vi "(SubVI)Scope_Log with Trigger.vi"(4 "Sampling Time":dbl format="%#_13g", 5 "Channel Settings":T1[](array[typedef]) {"Address" format="%04x"}, 6 "Log File Length":dbl=1.0 caption="Log File Length (sec.)" min=1.0, 7 "Init":bool, 8 "error in (no error)":errorcluster caption="에러 입력(에러 없음)", 9 "Trigger Setting":T2 {"Capture Delay (sec.)" min=0.0 max=5.0; "Pre-Trigger (sec.)" max=10.0}, 10 "Scope Data In":i16[][](array[numeric]), 11 "Path":path) -> (0 "error out":errorcluster caption="에러 출력", 3 "File Ref Out":refnum<file>)   [LabVIEW 2020]
uses:
  Controls/(Ctrl)Scope_Log_Trigger_Setting.ctl
  Controls/(Ctrl)Scope_Log_Trigger_Type.ctl
  Controls/(Ctrl)Scope_Log_Trigger_Edge.ctl
  Controls/(Ctrl)Scope_Log_Trigger_Edge_Slope.ctl
  Controls/(Ctrl)Scope_Log_Trigger_Window.ctl
  Controls/(Ctrl)Scope_Log_Trigger_Window_When.ctl
  Controls/(Ctrl)Scope_Log_Trigger_Mode.ctl
  Controls/(Ctrl)Scope_Settings.ctl
  Controls/(Ctrl)Scope_Log_Status.ctl
  000bd809-52dc-4150-b2e3-44c221babca0.vi
  03c6e600-b483-419d-b33d-b969c157e7dc.vi
panel:
  # "(SubVI)Scope_Log with Trigger.vi By hspark\n\nDescription : Scope 데이터를 csv 파일로 저장하는 VI. Trigger 기능 사용 시 Trigger를 찾는 연산도 수행함.\n\nInput : \n1. Path : 저장할 파일 경로\n2. Scope Data In : Scope 데이터 입력\n3. Trigger Setting : Trigger 설정 값 입력\n4. Init : True 입력 시 초기화\n5. Channel Settings : Header 생성을 위한 Scope 채널 설정 값 입력\n6. Log File Length : Log File의 최대 길이를 시간(초)으로 지정. 무한대 입력 시 파일을 끊지 않고 연속으로 저장함.\n7. Sampling Time : 시간 값 저장을 위한 Sampling Time(초) 입력\n\nOutput : \n1. File Ref Out : Scope 기능 종료 시 파일을 닫기 위한 파일 참조 출력\n\nLabVIEW Version : 2020 SP1 이상\n\nNote :\n\nUpdate : 2021.10.06"
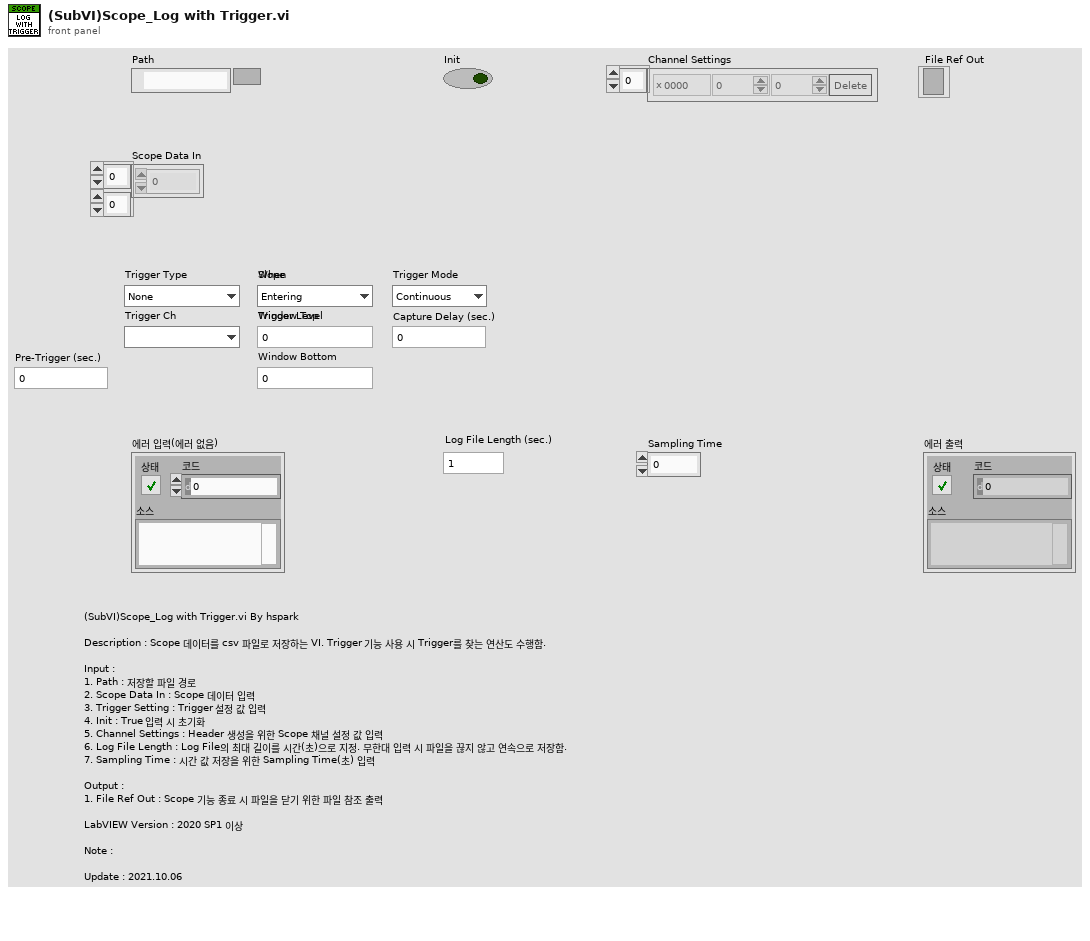
[diagram p1: front panel]
types:
  T1 = typedef "(Ctrl)Scope_Settings.ctl" = cluster{"Address":u16, "Scale":i32, "Offset":i32, "Delete":bool}
  T2 = typedef "(Ctrl)Scope_Log_Trigger_Setting.ctl" = cluster{"Trigger Type":T3, "Trigger Ch":u16, "Pre-Trigger (sec.)":dbl, "Trigger_Edge":T4, "Trigger_Window":T6, "Trigger Mode":T8, "Capture Delay (sec.)":dbl}
  T3 = typedef "(Ctrl)Scope_Log_Trigger_Type.ctl" = enum16{"None", "Edge", "Window"}
  T4 = typedef "(Ctrl)Scope_Log_Trigger_Edge.ctl" = cluster{"Slope":T5, "Trigger Level":i16}
  T5 = typedef "(Ctrl)Scope_Log_Trigger_Edge_Slope.ctl" = enum16{"Rising", "Falling"}
  T6 = typedef "(Ctrl)Scope_Log_Trigger_Window.ctl" = cluster{"When":T7, "Window Top":i16, "Window Bottom":i16}
  T7 = typedef "(Ctrl)Scope_Log_Trigger_Window_When.ctl" = enum16{"Entering", "Leaving"}
  T8 = typedef "(Ctrl)Scope_Log_Trigger_Mode.ctl" = enum16{"Continuous", "Capture"}
  T9 = typedef "(Ctrl)Scope_Log_Status.ctl" = enum16{"Waiting for Trigger", "Logging"}
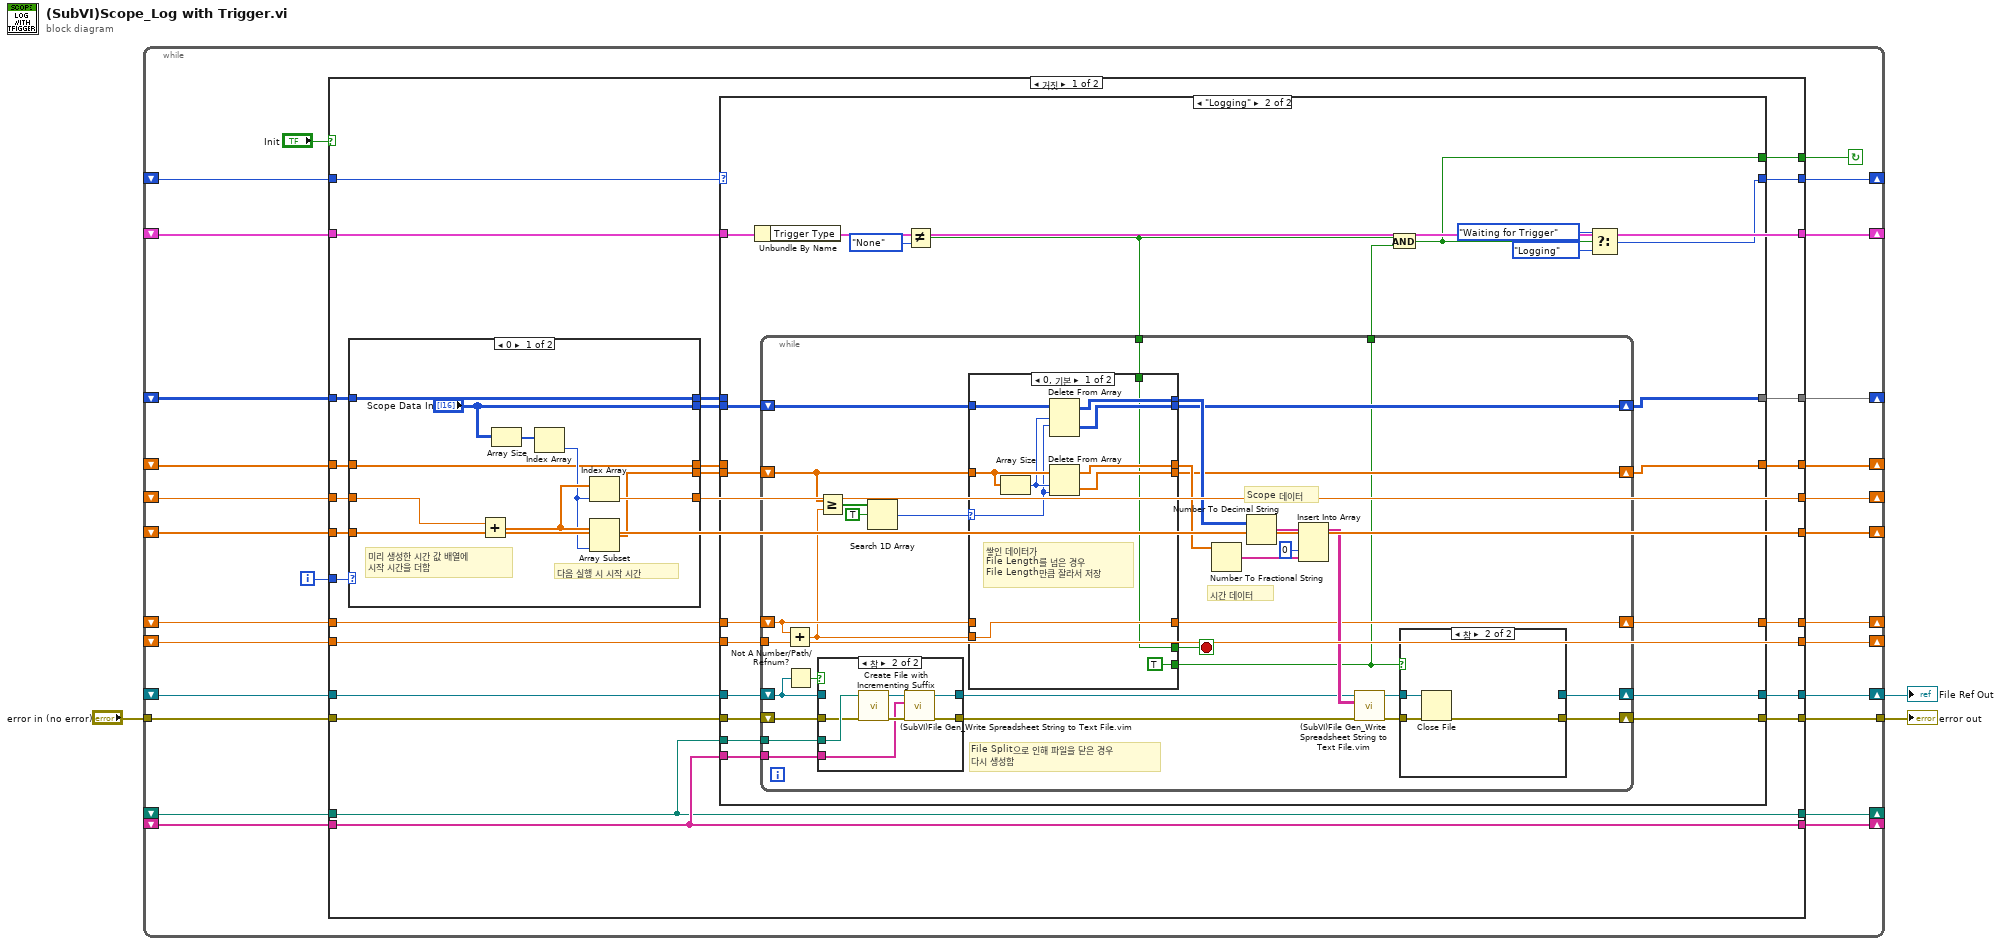
[diagram p0: block diagram]
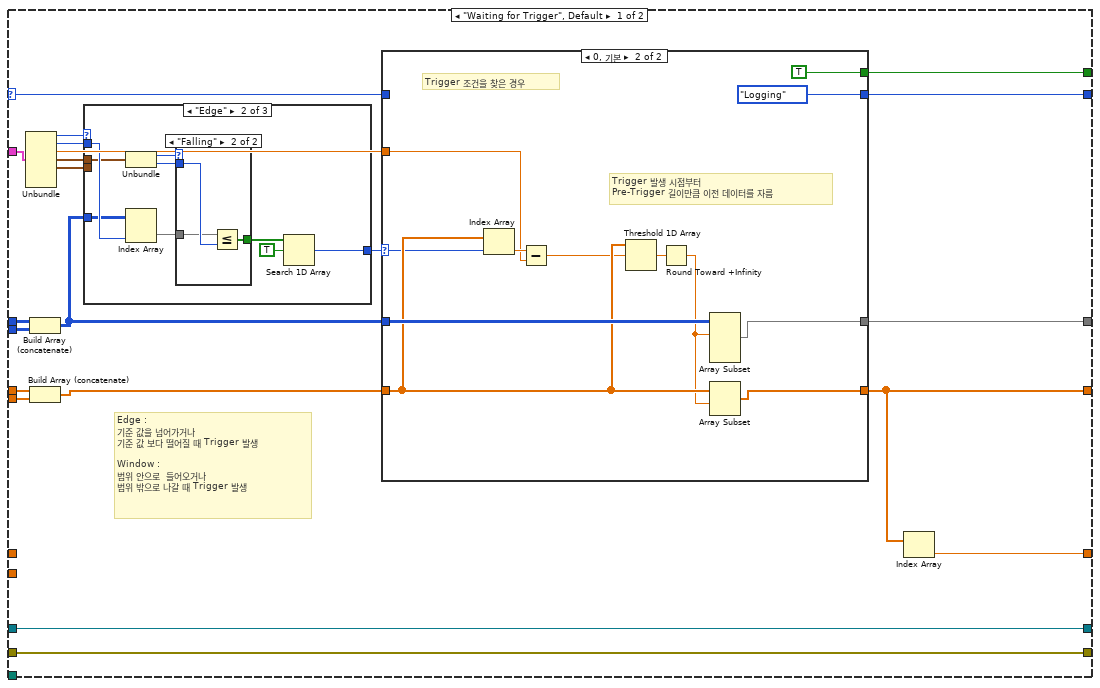
[diagram p3: hidden frame]
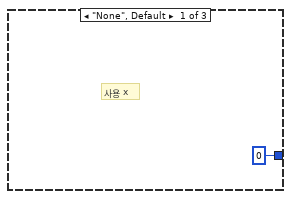
[diagram p4: hidden frame]
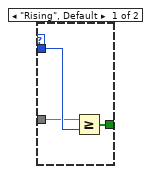
[diagram p5: hidden frame]
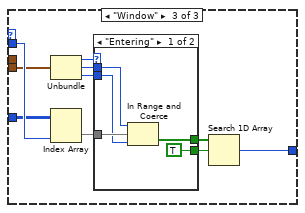
[diagram p6: hidden frame]
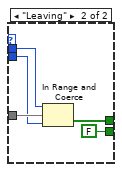
[diagram p7: hidden frame]
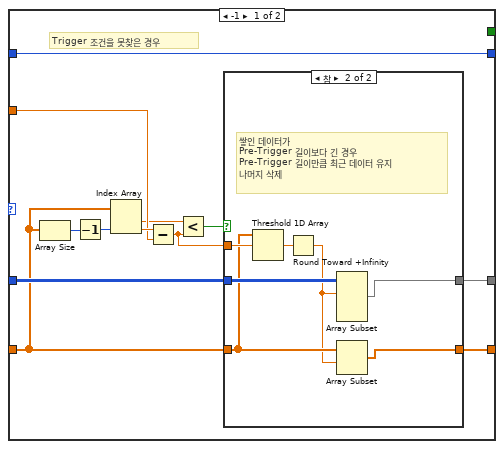
[diagram p8: hidden frame]
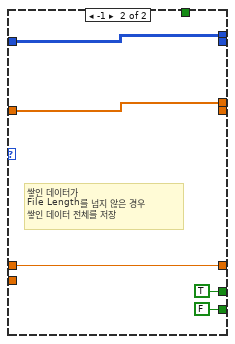
[diagram p12: hidden frame]
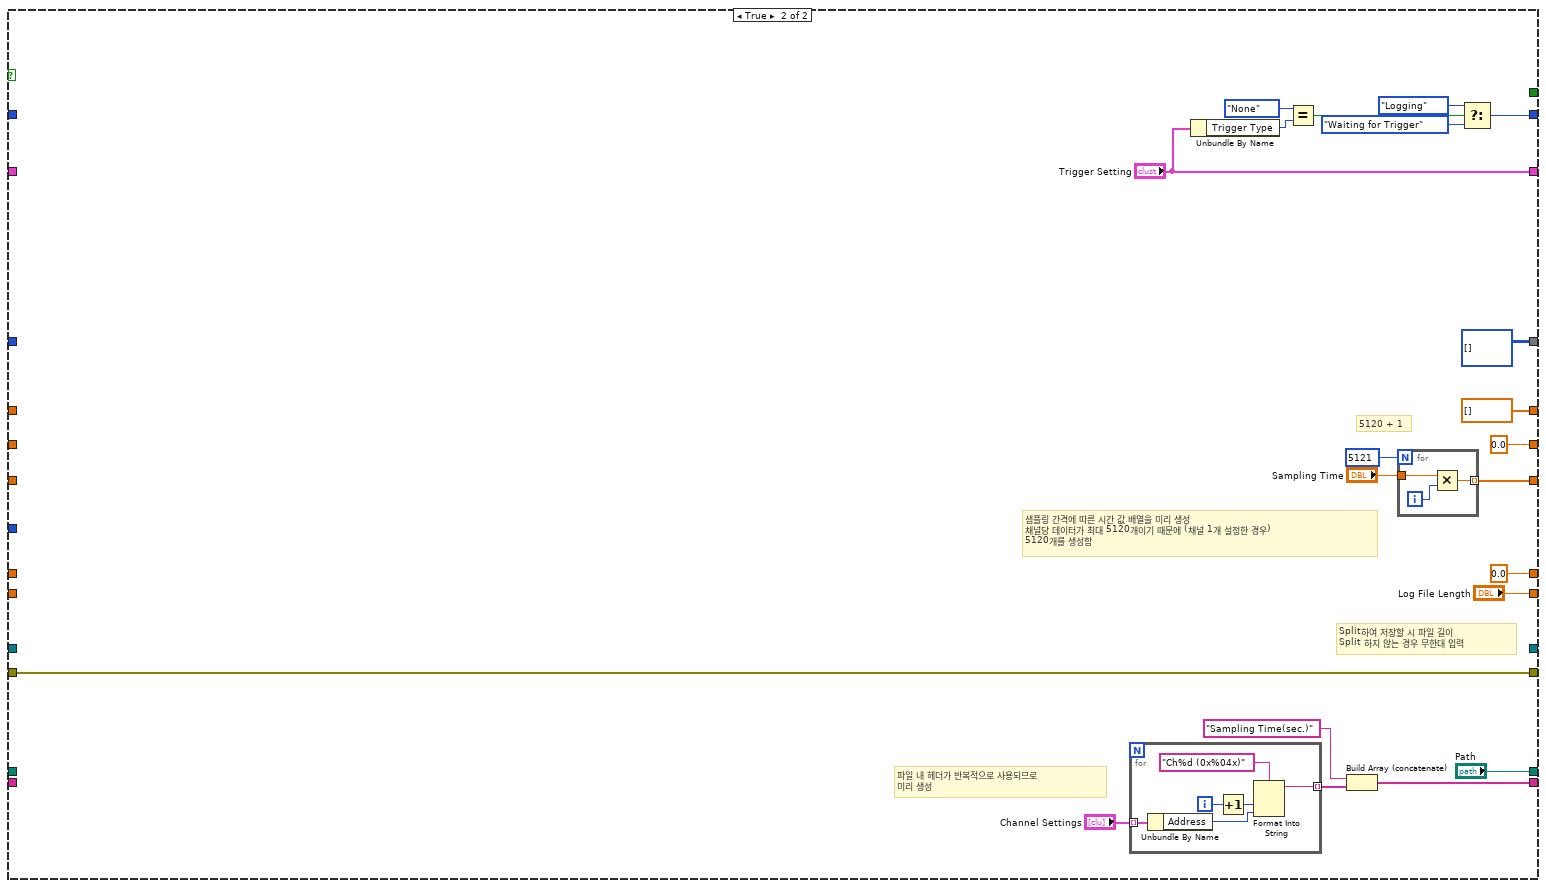
[diagram p13: hidden frame]
diagram:
  n1 = while {
    shift-right: [w30] -> _
    shift-left: _ -> [w28]
    shift-right: [w29] -> _
    shift-left: _ -> [w27]
    shift-right: [w25] -> _
    shift-left: _ -> [w24]
    shift-right: [w23] -> _
    shift-left: _ -> [w22]
    shift-right: [w20] -> _
    shift-left: _ -> [w19]
    shift-right: [w18] -> _
    shift-left: _ -> [w17]
    shift-right: [w15] -> w3
    shift-left: _ -> [w14]
    tunnel: "error in (no error)" -> [w13]
    tunnel: [w12] -> w1
    shift-right: [w11] -> _
    shift-left: _ -> [w10]
    shift-right: [w9] -> _
    shift-left: _ -> [w8]
    shift-right: [w7] -> _
    shift-left: _ -> [w6]
    shift-right: [w5] -> _
    shift-left: _ -> [w4]
    i -> [w16]
    stop <- w21 continue-if-true
    n2 = case shown="거짓" "Init" {
      tunnel: w24 -> [w47 _]
      tunnel: [w55 i16[][] [] ("Scope Data In")] -> w30
      tunnel: [w54 dbl[] [] ("Time Data In")] -> w29
      tunnel: w28 -> [w53 _]
      tunnel: w27 -> [w52 _]
      tunnel: [w47 "Trigger Setting"] -> w25
      tunnel: [w50 w256] -> w23
      tunnel: w22 -> [w51 _]
      tunnel: [w49 _] -> w21
      tunnel: [w46 0.0] -> w20
      tunnel: w19 -> [w48 _]
      tunnel: [w40 w250] -> w18
      tunnel: w17 -> [w40 _]
      tunnel: w16 -> [w43 _]
      tunnel: [w38 _] -> w15
      tunnel: w14 -> [w39 _]
      tunnel: w13 -> [w37 w242]
      tunnel: [w36 w242] -> w12
      tunnel: [w35 "Log File Length"] -> w11
      tunnel: w10 -> [w35 _]
      tunnel: [w33 0.0] -> w9
      tunnel: w8 -> [w34 _]
      tunnel: [w32 w244] -> w7
      tunnel: w6 -> [w32 _]
      tunnel: [w31 "Path"] -> w5
      tunnel: w4 -> [w31 _]
      frame False {
        n3 = case shown="0" w43 {
          tunnel: w53 -> [w59 w67]
          tunnel: w52 -> [w57 w66]
          tunnel: w48 -> [w64 w68]
          tunnel: [w61 w68] -> w46
          tunnel: w40 -> [w60 _]
          tunnel: [w57 _] -> w45
          tunnel: [w59 _] -> w44
          tunnel: ["Scope Data In" w67] -> w42
          tunnel: [w56 w66] -> w41
          frame 0 {
            # "다음 실행 시 시작 시간"
            # "미리 생성한 시간 값 배열에\n시작 시간을 더함"
            n4 = Add(x=w64, y=w60) -> (x+y=w63:dbl[])
            n5 = Array Size(array="Scope Data In") -> (size(s)=w65:i32[])
            n6 = Index Array(array=w65) -> (element=w62:i32)  [unwired: 1 in]
            n7 = Index Array(array=w63, index=w62) -> (element=w61:dbl)
            n8 = Array Subset(array=w63, length=w62) -> (w56:dbl[])  [unwired: 1 in]
          }
          frame 1, Default {
            # "Trigger 조건 찾은 후 Logging Status로 넘어온 경우\n(While Loop 반복인 경우)"
          }
        }
        n9 = case shown="\"Logging\"" w51 {
          selector: w51 -> [w84 _]
          tunnel: w47 -> [w89 w169]
          tunnel: [w85 w166] -> w55
          tunnel: [w69 w165] -> w54
          tunnel: w44 -> [w77 _]
          tunnel: w45 -> [w78 _]
          tunnel: [w80 w160] -> w50
          tunnel: [w79 w159] -> w49
          tunnel: w42 -> [w75 w180]
          tunnel: w41 -> [w73 w175]
          tunnel: w39 -> [w72 w179]
          tunnel: [w72 w178] -> w38
          tunnel: w37 -> [w71 w177]
          tunnel: [w71 w176] -> w36
          tunnel: w35 -> [_ w173]
          tunnel: w34 -> [_ w174]
          tunnel: [w70 w172] -> w33
          tunnel: w32 -> [_ w171]
          tunnel: w31 -> [_ w170]
          frame "Waiting for Trigger", Default {
            # "Edge : \n기준 값을 넘어가거나 \n기준 값 보다 떨어질 때 Trigger 발생\n\nWindow : \n범위 안으로  들어오거나 \n범위 밖으로 나갈 때 Trigger 발생"
            n10 = Unbundle(w89) -> ("Trigger Type"=w82:T3, "Trigger Ch"=w88:u16, "Pre-Trigger (sec.)"=w87:dbl, "Trigger_Edge"=w86:T4, "Trigger_Window"=w81:T6)  [unwired: 2 out]
            n11 = Build Array (concatenate)(w77, w75) -> (w76:i16[][])
            n12 = Build Array (concatenate)(w78, w73) -> (w74:dbl[])
            n13 = case shown="\"Edge\"" w82 {
              tunnel: w88 -> [_ w99 w115]
              tunnel: w86 -> [_ w98 _]
              tunnel: w76 -> [_ w97 w114]
              tunnel: [0 ("index of element") w94 w113] -> w83
              tunnel: w81 -> [_ _ w112]
              frame "None", Default {
                # "사용 x"
              }
              frame "Edge" {
                n14 = Unbundle(w98) -> ("Slope"=w91:T5, "Trigger Level"=w96:i16)
                n15 = Index Array(array=w97, index (col)=w99) -> (element=w95:i16[])  [unwired: 1 in]
                n16 = case shown="\"Falling\"" w91 {
                  tunnel: w96 -> [w102 w105]
                  tunnel: w95 -> [w101 w104]
                  tunnel: [w100 w103] -> w93
                  frame "Rising", Default {
                    n17 = Greater Or Equal?(x=w101, y=w102) -> (x >= y?=w100:bool[])
                  }
                  frame "Falling" {
                    n18 = Less Or Equal?(x=w104, y=w105) -> (x <= y?=w103:bool[])
                  }
                }
                n19 = Search 1D Array(1D array=w93, element=TRUE ("원소")) -> (index of element=w94:i32)  [unwired: 1 in]
              }
              frame "Window" {
                n20 = Unbundle(w112) -> ("When"=w106:T7, "Window Top"=w110:i16, "Window Bottom"=w109:i16)
                n21 = Index Array(array=w114, index (col)=w115) -> (element=w111:i16[])  [unwired: 1 in]
                n22 = case shown="\"Entering\"" w106 {
                  tunnel: w111 -> [w120 w125]
                  tunnel: w110 -> [w119 w124]
                  tunnel: w109 -> [w118 w123]
                  tunnel: [w117 w122] -> w108
                  tunnel: [TRUE FALSE] -> w107
                  frame "Entering" {
                    n23 = In Range and Coerce(upper limit=w119, x=w120, lower limit=w118) -> (In Range?=w117:bool[])  [unwired: 1 out]
                  }
                  frame "Leaving" {
                    n24 = In Range and Coerce(upper limit=w124, x=w125, lower limit=w123) -> (In Range?=w122:bool[])  [unwired: 1 out]
                  }
                }
                n25 = Search 1D Array(1D array=w108, element=w107) -> (index of element=w113:i32)  [unwired: 1 in]
              }
            }
            n26 = case shown="0, 기본" w83 {
              selector: w83 -> [_ w150]
              tunnel: w76 -> [w131 w156]
              tunnel: w74 -> [w130 w155]
              tunnel: w87 -> [w134 w157]
              tunnel: [w129 w154] -> w85
              tunnel: [w128 w153] -> w69
              tunnel: w84 -> [w126 _]
              tunnel: [w126 (Ctrl)Scope_Log_Status."Logging" ("f")] -> w80
              tunnel: [_ TRUE] -> w79
              frame -1 {
                # "Trigger 조건을 못찾은 경우"
                n27 = Array Size(array=w130) -> (size(s)=w137:i32)
                n28 = Decrement(x=w137) -> (x-1=w136:i32)
                n29 = Index Array(array=w130, index #2=w136) -> (element #1=w133:dbl, element #2=w135:dbl)  [unwired: 1 in]
                n30 = Subtract(x=w135, y=w134) -> (x-y=w127:dbl)
                n31 = Less?(x=w133, y=w127) -> (x < y?=w132:bool)
                n32 = case shown="참" w132 {
                  tunnel: w131 -> [w139 w145]
                  tunnel: w130 -> [w138 w144]
                  tunnel: [w139 w142] -> w129
                  tunnel: [w138 w141] -> w128
                  tunnel: w127 -> [_ w146]
                  frame False {
                    # "쌓인 데이터가 \nPre-Trigger 길이보다 짧은 경우"
                  }
                  frame True {
                    # "쌓인 데이터가 \nPre-Trigger 길이보다 긴 경우\nPre-Trigger 길이만큼 최근 데이터 유지\n나머지 삭제"
                    n33 = Threshold 1D Array(2:w146, 3:w144) -> (0:w143:dbl)  [unwired: 1 in]
                    n34 = Round Toward +Infinity(x=w143) -> (ceil(x): smallest int >= x=w140:dbl)
                    n35 = Array Subset(array=w145, index (row)=w140) -> (w142:i16[][])  [unwired: 3 in]
                    n36 = Array Subset(array=w144, index=w140) -> (w141:dbl[])  [unwired: 1 in]
                  }
                }
              }
              frame 0, Default {
                # "Trigger 발생 시점부터\nPre-Trigger 길이만큼 이전 데이터를 자름"
                # "Trigger 조건을 찾은 경우"
                n37 = Index Array(array=w155, index=w150) -> (element=w158:dbl)
                n38 = Subtract(x=w158, y=w157) -> (x-y=w152:dbl)
                n39 = Threshold 1D Array(2:w152, 3:w155) -> (0:w151:dbl)  [unwired: 1 in]
                n40 = Round Toward +Infinity(x=w151) -> (ceil(x): smallest int >= x=w147:dbl)
                n41 = Array Subset(array=w156, index (row)=w147) -> (w154:i16[][])  [unwired: 3 in]
                n42 = Array Subset(array=w155, index=w147) -> (w153:dbl[])  [unwired: 1 in]
              }
            }
            n43 = Index Array(array=w69) -> (element=w70:dbl)  [unwired: 1 in]
          }
          frame "Logging" {
            n44 = Unbundle By Name(w169) -> ("Trigger Type"=w168:T3)
            n45 = Not Equal?(x=w168, y=(Ctrl)Scope_Log_Trigger_Type."None") -> (x != y?=w164:bool)
            n46 = while {
              shift-right: [w191] -> w176
              shift-left: w177 -> [w185]
              shift-right: [w192] -> w178
              shift-left: w179 -> [w186]
              shift-right: [w196] -> w172
              shift-left: w174 -> [w197]
              tunnel: w173 -> [w205]
              shift-right: [w199] -> w166
              shift-left: w180 -> [w203]
              shift-right: [w198] -> w165
              shift-left: w175 -> [w202]
              tunnel: w171 -> [w181]
              tunnel: w170 -> [w182]
              tunnel: w164 -> [w189]
              tunnel: [w188] -> w163
              stop <- w195 stop-if-true
              # "시간 데이터"
              # "Scope 데이터"
              # "File Split으로 인해 파일을 닫은 경우\n다시 생성함"
              n47 = Add(x=w197, y=w205) -> (x+y=w190:dbl)
              n48 = Not A Number/Path/Refnum?(number/path/refnum=w186) -> (NaN/Path/Refnum?=w187:bool)
              n49 = Greater Or Equal?(x=w202, y=w190) -> (x >= y?=w207:bool[])
              n50 = case shown="참" w187 {
                tunnel: w186 -> [w213 _]
                tunnel: w185 -> [w212 w216]
                tunnel: [w213 w214] -> w184
                tunnel: [w212 w215] -> w183
                tunnel: w182 -> [_ w218]
                tunnel: w181 -> [_ w217]
                frame False {
                }
                frame True {
                  n51 = call <vilib>:"Create File with Incrementing Suffix.vi"("error in (no error)"=w216, "file path"=w218) -> ("error out"=w219:errorcluster, "refnum out"=w220:refnum<file>)  [unwired: 7 in, 1 out]
                  n52 = call "(SubVI)File Gen_Write Spreadsheet String to Text File.vim"("Error In"=w219, "Array"=w217, "File Ref In"=w220) -> ("Error Out"=w215:errorcluster, "File Ref Out"=w214:refnum<file>)  [unwired: 7 in]
                }
              }
              n53 = Search 1D Array(1D array=w207, element=TRUE ("원소")) -> (index of element=w204:i32)  [unwired: 1 in]
              n54 = case shown="0, 기본" w204 {
                selector: w204 -> [w233 _]
                tunnel: w203 -> [w236 w241]
                tunnel: w202 -> [w235 w240]
                tunnel: [w231 w241] -> w201
                tunnel: [w229 w240] -> w200
                tunnel: [w226 TRUE] -> w195
                tunnel: [w232 _] -> w199
                tunnel: [w230 _] -> w198
                tunnel: w197 -> [_ w239]
                tunnel: [w228 w239] -> w196
                tunnel: w190 -> [w228 _]
                tunnel: w189 -> [w226 _]
                tunnel: [TRUE FALSE] -> w188
                frame 0, Default {
                  # "쌓인 데이터가\nFile Length를 넘은 경우\nFile Length만큼 잘라서 저장"
                  n55 = Array Size(array=w235) -> (size(s)=w234:i32)
                  n56 = Delete From Array(array=w236, length=w234, index (row)=w233) -> (deleted portion=w232:i16[][], array with subset deleted=w231:i16[][])  [unwired: 1 in]
                  n57 = Delete From Array(array=w235, length=w234, index=w233) -> (deleted portion=w230:dbl[], array with subset deleted=w229:dbl[])
                }
                frame -1 {
                  # "쌓인 데이터가\nFile Length를 넘지 않은 경우\n쌓인 데이터 전체를 저장"
                }
              }
              n58 = Number To Fractional String(number=w200) -> (F-format string=w211:string[])  [unwired: 3 in]
              n59 = Number To Decimal String(number=w201) -> (decimal integer string=w208:string[][])  [unwired: 1 in]
              n60 = Insert Into Array(array=w208, index (col)=0 ("비활성화된 인덱스 (열)"), new element=w211) -> (w210:string[][])  [unwired: 1 in]
              n61 = call "(SubVI)File Gen_Write Spreadsheet String to Text File.vim"("Error In"=w183, "Array"=w210, "File Ref In"=w184) -> ("Error Out"=w193:errorcluster, "File Ref Out"=w194:refnum<file>)  [unwired: 7 in]
              n62 = case shown="참" w188 {
                tunnel: w194 -> [w222 w224]
                tunnel: w193 -> [w221 w225]
                tunnel: [w222 _] -> w192
                tunnel: [w221 w223] -> w191
                frame False {
                }
                frame True {
                  n63 = Close File(refnum=w224, error in=w225) -> (error out=w223:errorcluster)  [unwired: 1 out]
                }
              }
            }
            n64 = And(x=w164, y=w163) -> (x .and. y?=w159:bool)
            n65 = Select(t=(Ctrl)Scope_Log_Status."Waiting for Trigger" ("f"), s=w159, f=(Ctrl)Scope_Log_Status."Logging") -> (s? t:f=w160:T9)
          }
        }
      }
      frame True {
        # "Split하여 저장할 시 파일 길이\nSplit 하지 않는 경우 무한대 입력"
        # "샘플링 간격에 따른 시간 값 배열을 미리 생성\n채널당 데이터가 최대 5120개이기 때문에 (채널 1개 설정한 경우)\n5120개를 생성함"
        # "파일 내 헤더가 반복적으로 사용되므로\n미리 생성"
        # "5120 + 1"
        n66 = for {
          tunnel: "Channel Settings" -> [w268] mode=indexing
          tunnel: [w263] -> w248 mode=indexing
          i -> [w267]
          n67 = Unbundle By Name(w268) -> ("Address"=w264:u16)
          n68 = Increment(x=w267) -> (x+1=w265:i32)
          n69 = Format Into String(format string="Ch%d (0x%04x)" ("포맷 문자열"), w265, w264) -> (resulting string=w263:string)  [unwired: 2 in, 1 out]
        }
        n70 = Unbundle By Name("Trigger Setting") -> ("Trigger Type"=w261:T3)
        n71 = Equal?(x=(Ctrl)Scope_Log_Trigger_Type."None", y=w261) -> (x = y?=w259:bool)
        n72 = Build Array (concatenate)("Sampling Time(sec.)" ("배열"), w248) -> (w244:string[])
        n73 = for {
          N: 5121 -> [_]
          tunnel: "Sampling Time" -> [w270]
          tunnel: [w269] -> w250 mode=indexing
          i -> [w271]
          n74 = Multiply(x=w270, y=w271) -> (x*y=w269:dbl)
        }
        n75 = Select(t=(Ctrl)Scope_Log_Status."Logging", s=w259, f=(Ctrl)Scope_Log_Status."Waiting for Trigger") -> (s? t:f=w256:T9)
      }
    }
  }
  "error out" <- w1
  "File Ref Out" <- w3
